vi "ConfigClock.vi"(8 "error in (no error)":errorcluster, 11 "NiPxi6733 in":refnum<class "NiPxi6733.lvclass">) -> (0 "error out":errorcluster, 3 "NiPxi6733 out":refnum<class "NiPxi6733.lvclass">)   [LabVIEW 2014, in "FgenPlugins.lvlib" / "NiPxi6733.lvclass"]
uses:
  NiPxi6733.lvclass
  NiPxi6733.lvclass/NiPxi6733.ctl
  FgenPluginBaseClass/FgenPluginsBase.lvclass/FgenPluginsBase.ctl
  Accessors/Read Timebase.vi
  Accessors/Read SampleRate.vi
  FgenPluginBaseClass/Accessors/Read Channels.vi
  <vilib>/DAQmx/configure/timing.llb/DAQmx Timing (Sample Clock).vi
  <resource>/objmgr/daqmx.rc
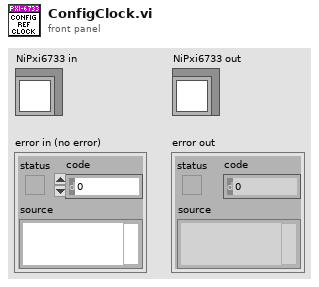
[diagram p1: front panel]
types:
  T1 = typedef "FgenPlugins.lvlib/NiPxi6733.lvclass/Timebase.ctl" = cluster{"source":string, "rate":dbl}
  T2 = typedef "FgenPlugins.lvlib/Channel.ctl" = cluster{"Name":string, "Enabled":bool, "Operation":enum16{"Continuous", "Burst"}, "Impedance (50)":dbl, "Handle":string, "Connected":bool, "Mode (Function)":enum16{"Function", "Arbitrary", "Sequence"}}
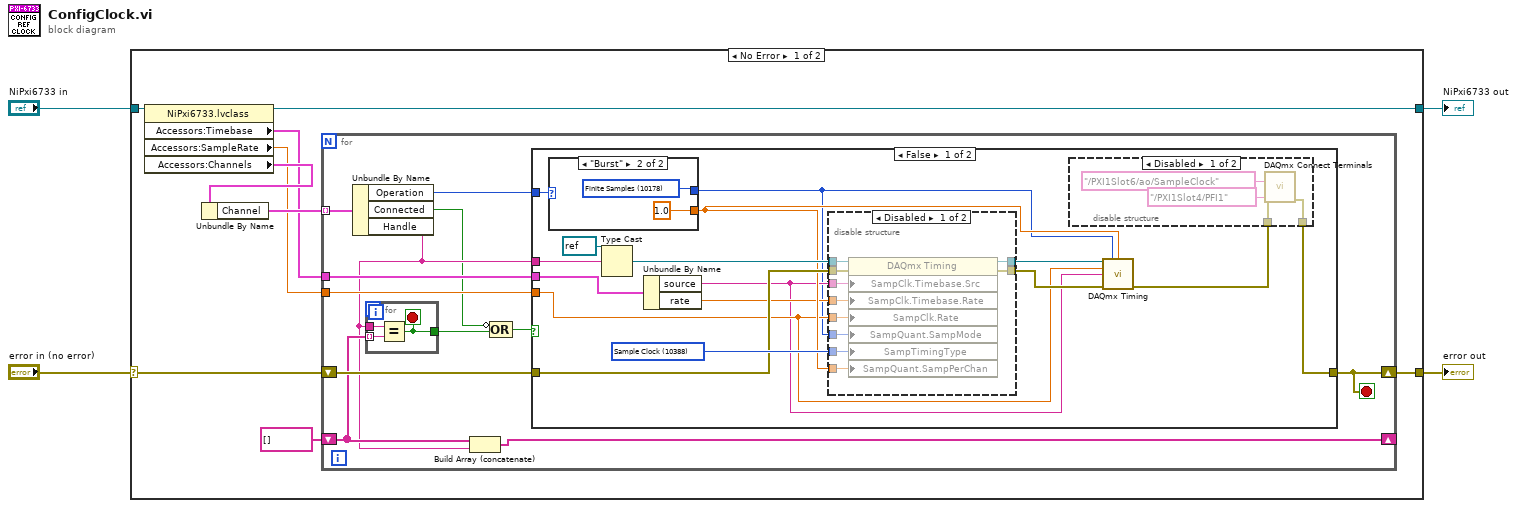
[diagram p0: block diagram]
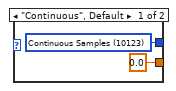
[diagram p4: hidden frame]
diagram:
  n1 = case shown="No Error" "error in (no error)" {
    selector: "error in (no error)" -> [w12 w68]
    tunnel: [w9 w68] -> w3
    tunnel: [w5 w67] -> w1
    tunnel: "NiPxi6733 in" -> [w13 w67]
    frame No Error {
      n2 = property class="NiPxi6733.lvclass"(reference=w13) -> (reference out=w5:refnum<class "NiPxi6733.lvclass">, "Accessors:Timebase"=w6:T1, "Accessors:SampleRate"=w7:dbl, "Accessors:Channels"=w8:cluster{"Count":u16, "Channel":T2[]})  [unwired: 1 in, 1 out]
      n3 = Unbundle By Name(w8) -> ("Channel"=w11:T2[])
      n4 = for {
        shift-right: [w22] -> w9
        shift-left: w12 -> [w24]
        tunnel: w11 -> [w19] mode=indexing
        tunnel: w7 -> [w23]
        shift-right: [w20] -> _
        shift-left: string[] [] -> [w21]
        tunnel: w6 -> [w18]
        stop <- w22 stop-if-true
        n5 = Unbundle By Name(w19) -> ("Operation"=w25:enum16{"Continuous", "Burst"}, "Connected"=w15:bool, "Handle"=w17:string)
        n6 = for {
          tunnel: w21 -> [w66] mode=indexing
          tunnel: w17 -> [w65]
          tunnel: [w64] -> w16
          stop <- w64 stop-if-true
          n7 = Equal?(x=w65, y=w66) -> (x = y?=w64:bool)
        }
        n8 = Build Array (concatenate)(w21, w17) -> (w20:string[])
        n9 = Compound Arithmetic op=OR(invert w15, w16) -> (w14:bool)
        n10 = case shown="False" w14 {
          tunnel: w25 -> [w41 _]
          tunnel: w24 -> [w35 w63]
          tunnel: w17 -> [w39 _]
          tunnel: w23 -> [w28 _]
          tunnel: [w34 w63] -> w22
          tunnel: w18 -> [w36 _]
          frame False {
            w37 = 10388 items=["Sample Clock"=10388, "Burst Handshake"=12548, "Handshake"=10389, "Implicit"=10451, "On Demand"=10390, "Change Detection"=12504, "Pipelined Sample Clock"=14668] ("SampTimingType")
            n11 = case shown="\"Burst\"" w41 {
              tunnel: [w60 w62] -> w26
              tunnel: [0.0 1.0] -> w30
              frame "Continuous", Default {
                w60 = 10123 items=["Finite Samples"=10178, "Continuous Samples"=10123, "Hardware Timed Single Point"=12522] ("SampQuant.SampMode")
              }
              frame "Burst" {
                w62 = 10178 items=["Finite Samples"=10178, "Continuous Samples"=10123, "Hardware Timed Single Point"=12522] ("SampQuant.SampMode")
              }
            }
            n12 = Type Cast(type=refnum<k21> refnum ("DAQmx Task Name"), x=w39) -> (*(type *) &x=w38:refnum<k21>)
            n13 = Unbundle By Name(w36) -> ("source"=w27:string, "rate"=w29:dbl)
            n14 = disable-structure shown="Disabled" {
              disable-tunnel: w38 -> [w51 w53]
              disable-tunnel: w37 -> [w50 _]
              disable-tunnel: w35 -> [w49 w52]
              disable-tunnel: [w48 w52] -> w33
              disable-tunnel: [w47 w53] -> w31
              disable-tunnel: w26 -> [w46 _]
              disable-tunnel: w30 -> [w45 _]
              disable-tunnel: w29 -> [w44 _]
              disable-tunnel: w28 -> [w43 _]
              disable-tunnel: w27 -> [w42 _]
              frame Disabled {
                n15 = property class="DAQmx Timing"(reference=w51, error in=w49, "SampClk.Timebase.Src"=w42, "SampClk.Timebase.Rate"=w44, "SampClk.Rate"=w43, "SampQuant.SampMode"=w46, "SampTimingType"=w50, "SampQuant.SampPerChan"=w45) -> (reference out=w47:refnum<k21>, error out=w48:errorcluster)
              }
              frame Enabled {
              }
            }
            n16 = call-poly <vilib>:"DAQmx Timing.vi"("task/channels in"=w31, "sample mode"=w26, "samples per channel"=w30, "rate"=w28, "source"=w27, "error in"=w33) -> ("error out"=w32:errorcluster)  [unwired: 8 in, 1 out]
            n17 = disable-structure shown="Disabled" {
              disable-tunnel: w32 -> [w57 w58]
              disable-tunnel: [w56 w58] -> w34
              frame Disabled {
                n18 = call <vilib>:"DAQmx Connect Terminals.vi"("source terminal"=tag "/PXI1Slot6/ao/SampleClock", "destination terminal"=tag "/PXI1Slot4/PFI1", "error in"=w57) -> ("error out"=w56:errorcluster)  [unwired: 12 in]
              }
              frame Enabled {
              }
            }
          }
          frame True {
          }
        }
      }
    }
    frame Error {
    }
  }
  "error out" <- w3
  "NiPxi6733 out" <- w1
